vi "ErrorCaseNames.vi"(6 "error in":errorcluster) -> (0 "error out":errorcluster, 4 "Error":string, 5 "No Error":string)   [LabVIEW 2014, in "Raspberry Pi Compatible Compiler for LabVIEW.lvlib" / "CaseStructure.lvclass"]
uses:
  CaseStructure.lvclass
  <vilib>/Utility/traverseref.llb/TRef TravTarget.ctl
  <vilib>/regexp/Match Regular Expression.xnode
  <vilib>/Utility/traverseref.llb/VI Scripting - Traverse.lvlib
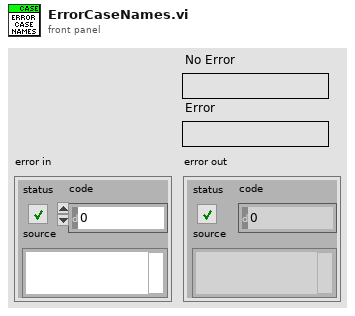
[diagram p1: front panel]
types:
  T1 = typedef "TRef TravTarget.ctl" = enum16{"FP", "BD", "Other"}
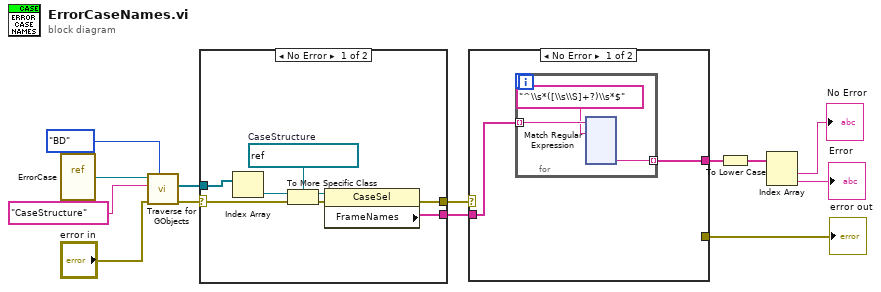
[diagram p0: block diagram]
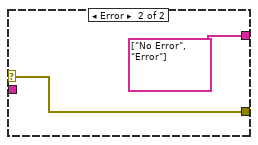
[diagram p2: hidden frame]
diagram:
  n1 = vi-ref "ErrorCase.vi"() -> (w8:refnum<vi>)
  n2 = call <vilib>:"Traverse for GObjects.vi"("Traverse Target"=TRef_TravTarget."BD", "error in (no error)"="error in", "Class Name"="CaseStructure", "VI Refnum"=w8) -> ("error out"=w9:errorcluster, "References"=w10:refnum<vi>[])  [unwired: 4 in, 2 out]
  n3 = case shown="No Error" w9 {
    selector: w9 -> [w19 w22]
    tunnel: w10 -> [w21 _]
    tunnel: [w15 w22] -> w11
    tunnel: [w14 _] -> w12
    frame No Error {
      w18 = refnum<vi> refnum  # CaseStructure
      n4 = Index Array(array=w21) -> (element=w20:refnum<vi>)  [unwired: 1 in]
      n5 = To More Specific Class(target class=w18, reference=w20, error in=w19) -> (specific class reference=w17:refnum<vi>, error out=w16:errorcluster)
      n6 = property class="CaseSel"(reference=w17, error in=w16) -> (error out=w15:errorcluster, "FrameNames"=w14:string[])  [unwired: 1 out]
    }
    frame Error {
    }
  }
  n7 = case shown="No Error" w11 {
    selector: w11 -> [_ w144]
    tunnel: w12 -> [w24 _]
    tunnel: [w23 string[] ["No Error", "Error"] ("FrameNames")] -> w13
    tunnel: [_ w144] -> w1
    frame No Error {
      n8 = for {
        tunnel: w24 -> [w27] mode=indexing
        tunnel: [w26] -> w23 mode=indexing
        n9 = xnode "Match Regular Expression"("input string"=w27, "regular expression"="^\\s*([\\s\\S]+?)\\s*$") -> ("submatch 1"=w26:string)  [unwired: 4 in, 5 out]
      }
    }
    frame Error {
    }
  }
  "error out" <- w1
  n10 = To Lower Case(string=w13) -> (all lower case string=w5:string[])
  n11 = Index Array(array=w5) -> (element #1=→"No Error":string, element #2=→"Error":string)  [unwired: 2 in]
